vi "rescaleImage.vi"(11 "Refnum in":T1) -> (2 "bin":i32, 3 "Refnum out":T1)   [LabVIEW 2011]
uses:
  IMAQ Image.ctl
  NI_Vision_Development_Module.lvlib
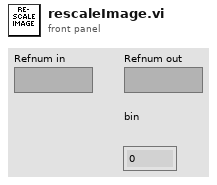
[diagram p1: front panel]
types:
  T1 = typedef "IMAQ Image.ctl" = refnum<image>
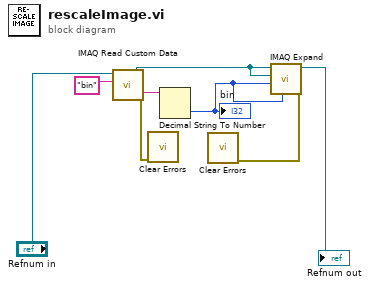
[diagram p0: block diagram]
diagram:
  n1 = call "IMAQ Read Custom Data"("Key"="bin", "Image"="Refnum in") -> ("error out"=w8:errorcluster, "Custom Data Out"=w2:string, "Image (duplicate)"=w7:T1)  [unwired: 7 in]
  n2 = call "Clear Errors.vi"("error in (no error)"=w8) -> ()  [unwired: 6 in, 1 out]
  n3 = Decimal String To Number(string=w2) -> (number=w6:i32)  [unwired: 2 in, 1 out]
  "bin" <- w6
  n4 = call "IMAQ Expand"("Y Duplication Step"=w6, "X Duplication Step"=w6, "Image Dst"=w7, "Image Src"=w7) -> ("error out"=w5:errorcluster, "Image Dst Out"=→"Refnum out":T1)  [unwired: 6 in]
  n5 = call "Clear Errors.vi"("error in (no error)"=w5) -> ()  [unwired: 6 in, 1 out]
